vi "DSC TSV Process Path.vi"(8 "error in (no error)":errorcluster, 11 "path in":path=path "G:/.shortcut-targets-by-id/1WDr4dR83sFDxMqrJrBnKdnzPXtLPCjmG/Database Data/Cryostation/Platform Temperature (K)/2020") -> (0 "error out":errorcluster, 2 "process path":path=path "G:/.shortcut-targets-by-id/1WDr4dR83sFDxMqrJrBnKdnzPXtLPCjmG/Database Data/PROCESSED/Cryostation/Platform Temperature (K)/2020", 3 "path out":path=path "G:/.shortcut-targets-by-id/1WDr4dR83sFDxMqrJrBnKdnzPXtLPCjmG/Database Data/Cryostation/Platform Temperature (K)/2020")   [LabVIEW 2019, in "LV-Data.PGSQL.lvclass"]
uses:
  LV-Data.PGSQL.lvclass
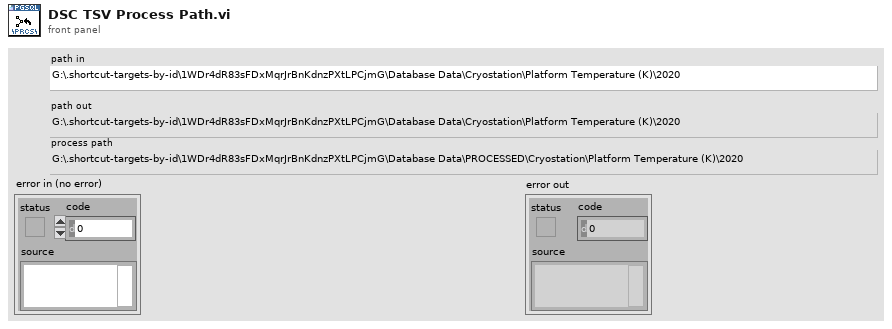
[diagram p1: front panel]
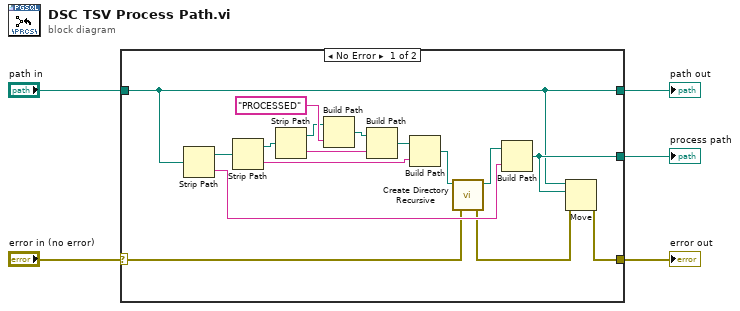
[diagram p0: block diagram]
diagram:
  n1 = case shown="No Error" "error in (no error)" {
    selector: "error in (no error)" -> [w8 w23]
    tunnel: [w10 _] -> w5
    tunnel: "path in" -> [w7 w22]
    tunnel: [w6 w23] -> w3
    tunnel: [w7 w22] -> w1
    frame No Error {
      n2 = Strip Path(path=w7) -> (stripped path=w13:path, name=w21:string)
      n3 = Strip Path(path=w13) -> (stripped path=w14:path, name=w20:string)
      n4 = Strip Path(path=w14) -> (stripped path=w15:path, name=w19:string)
      n5 = Build Path(base path=w15, name or relative path="PROCESSED") -> (appended path=w16:path)
      n6 = Build Path(base path=w16, name or relative path=w19) -> (appended path=w17:path)
      n7 = Build Path(base path=w17, name or relative path=w20) -> (appended path=w12:path)
      n8 = call <vilib>:"Create Directory Recursive.vi"("error in (no error)"=w8, "directory"=w12) -> ("error out"=w9:errorcluster, "directory copy"=w11:path)  [unwired: 3 in, 1 out]
      n9 = Build Path(base path=w11, name or relative path=w21) -> (appended path=w10:path)
      n10 = Move(source path=w7, error in=w9, 10:w10) -> (error out=w6:errorcluster)  [unwired: 2 in, 2 out]
    }
    frame Error {
    }
  }
  "process path" <- w5
  "path out" <- w1
  "error out" <- w3
